vi "Sequence.Test.Print.Ready.vi"(10 "Data in":T8, 11 "Code in":T1={"Ready"=FALSE, "DoubleOrder"=FALSE, "OrderDone"=FALSE, "AllowSingleSlot"=FALSE, "TunedA"=FALSE, "TunedB"=FALSE, "CheckDM"=FALSE, "ThresholdA"=0, "ThresholdB"=0, "Plate"=enum."Wabco", "ImgPath"=path "", "Variant"={"State"=enum."Init", "ImgPath"=path "", "WabcoPlate"="", "WabcoProduct"="", "ClientProduct"="", "ClientPlate"="", "TotalQuantity"=0, "OrderQuantity"=0, "Serial"=0, "Wabco"={"LaserJob"="", "AdditionalTxt"="037", "FactoryCode"="", "RevID"=0, "ForkID"=0, "FailuresLimit"=0, "GlobalCnt"=0, "Bank"=0, "SerialFormat"=enum."6 dig", "CoordA"={"X"=0.0, "Y"=0.0, "Angle"=0.0}, "CoordB"={"X"=0.0, "Y"=0.0, "Angle"=0.0}, "DMCconfig"=0}, "Client"={"LaserJob"="", "AdditionalTxt"="", "FactoryCode"="037", "RevID"=0, "ForkID"=0, "FailuresLimit"=0, "GlobalCnt"=0, "Bank"=0, "SerialFormat"=enum."6 dig", "CoordA"={"X"=0.0, "Y"=0.0, "Angle"=0.0}, "CoordB"={"X"=0.0, "Y"=0.0, "Angle"=0.0}, "DMCconfig"=0}}}) -> (1 "Print B":bool, 2 "Print A":bool)   [LabVIEW 2016]
uses:
  Sequence.Test.Status.ctl
  Sequence.Slot.StatusData.ctl
  Sequence.Test.Unload.Status.ctl
  Sequence.Prod.StatusData.ctl
  Sequence.Step.Status.ctl
  Sequence.Test.BreakReason.ctl
  Sequence.Code.Sets.ctl
  Sequence.PlateType.ctl
  Logger/Logger.Variant.Sets.ctl
  Station/Station.Changeover.State.vi
  Station/Station.Plate.Properties.ctl
  Sequence.Code.SerialFormat.ctl
  Drivers/V7310/LowLevel/V7310.Job.Sets.ctl
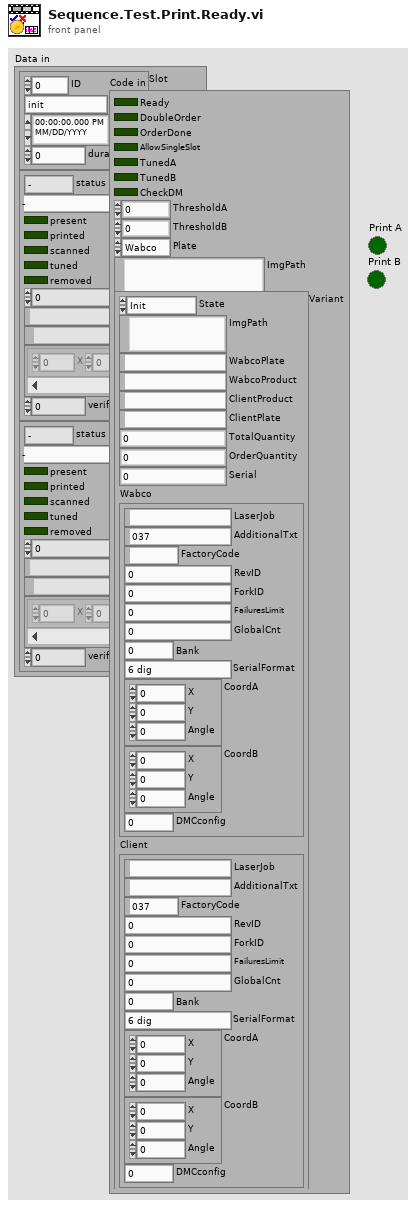
[diagram p1: front panel]
types:
  T1 = typedef "Sequence.Code.Sets.ctl" = cluster{"Ready":bool, "DoubleOrder":bool, "OrderDone":bool, "AllowSingleSlot":bool, "TunedA":bool, "TunedB":bool, "CheckDM":bool, "ThresholdA":u8, "ThresholdB":u8, "Plate":T2, "ImgPath":path, "Variant":T3}
  T2 = typedef "Sequence.PlateType.ctl" = enum16{"Wabco", "Client"}
  T3 = typedef "Logger.Variant.Sets.ctl" = cluster{"State":T4, "ImgPath":path, "WabcoPlate":string, "WabcoProduct":string, "ClientProduct":string, "ClientPlate":string, "TotalQuantity":u16, "OrderQuantity":u16, "Serial":i32, "Wabco":T5, "Client":T5}
  T4 = typedef "Station.Changeover.State.vi" = enum16{"Init", "Scaning", "NOK", "Wait for ack", "Ready"}
  T5 = typedef "Station.Plate.Properties.ctl" = cluster{"LaserJob":string, "AdditionalTxt":string, "FactoryCode":string, "RevID":u8, "ForkID":u8, "FailuresLimit":u16, "GlobalCnt":i32, "Bank":u8, "SerialFormat":T6, "CoordA":T7, "CoordB":T7, "DMCconfig":i32}
  T6 = typedef "Sequence.Code.SerialFormat.ctl" = enum8{"", "6 dig", "7 dig"}
  T7 = typedef "V7310.Job.Sets.ctl" = cluster{"X":dbl, "Y":dbl, "Angle":dbl}
  T8 = typedef "Sequence.Test.Status.ctl" = cluster{"Slot":T9, "A":T11, "B":T11}
  T9 = typedef "Sequence.Slot.StatusData.ctl" = cluster{"ID":i32, "Unload":T10, "TS":timestamp, "duration":u32}
  T10 = typedef "Sequence.Test.Unload.Status.ctl" = enum16{"init", "check NOK", "check OK", "wait on NOK", "wait on OK", "wait on Unload", "done"}
  T11 = typedef "Sequence.Prod.StatusData.ctl" = cluster{"status":T12, "pause":T13, "present":bool, "printed":bool, "scanned":bool, "tuned":bool, "removed":bool, "serial":i32, "code":string, "path":path, "corners":cluster{"X":i32, "Y":i32}[], "verification":u8}
  T12 = typedef "Sequence.Step.Status.ctl" = enum16{"-", "Pending", "Running", "Skipped", "Passed", "Failed", "Done", "Error", "Aborted", "Stopped"}
  T13 = typedef "Sequence.Test.BreakReason.ctl" = enum16{"-", "NOK container", "OK container", "Rev empty", "Rev missing", "Rev wrong", "Fork missing", "Fork wrong", "NOK limit", "Unload failure", "Single slot", "Part done", "Err: Prod move work", "Err: Prod move home", "Err: Prod lift work", "Err: Prod lift home", "Err: Prod Arm Work", "Err: Prod Arm NOK", "Err: Prod Arm OK", "Err: Prod NOK suck", "Err: Prod NOK drop", "Err: Prod OK missing", "Err: Prod OK suck", "Err: Prod OK drop"}
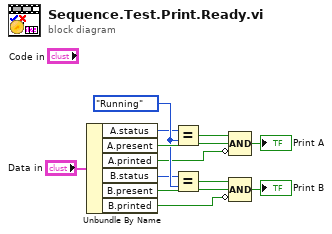
[diagram p0: block diagram]
diagram:
  w10 = Sequence.Step.Status."Running" ("y")
  n1 = Unbundle By Name("Data in") -> ("A.status"=w7:T12, "A.present"=w12:bool, "A.printed"=w4:bool, "B.status"=w6:T12, "B.present"=w11:bool, "B.printed"=w3:bool)
  n2 = Equal?(x=w7, y=w10) -> (x = y?=w9:bool)
  n3 = Equal?(x=w6, y=w10) -> (x = y?=w8:bool)
  n4 = Compound Arithmetic op=AND(w9, w12, invert w4) -> (→"Print A":bool)
  n5 = Compound Arithmetic op=AND(w8, w11, invert w3) -> (→"Print B":bool)
